vi "AssertVIExecCore.vi"(0 "VI Reference In":refnum<vi>, 1 "Label":string, 3 "Assert Only? (F)":bool, 5 "Execution:State":T2(array[ring]), 11 "Error In":errorcluster, 12 "Assert Interval(10 ms)":u32=10, 13 "Timeout(5 sec)":dbl=5.0) -> (4 "VI Reference Out":refnum<vi>, 6 "Asserted Value":T1(ring), 15 "Error Out":errorcluster)   [LabVIEW 2016, in "Drona.lvlib" / "AssertVI.lvlib"]
doc: "Asserts the execution state of the VI.\nThe input control name is given as a string , incase of path, use delimiters inbetween the path."
uses:
  AssertVI.lvlib
  <vilib>/addons/_JKI Toolkits/Caraya/classes/Assert/Assert True.vi
  <vilib>/addons/_JKI Toolkits/Caraya/classes/Assert/Assert.lvclass
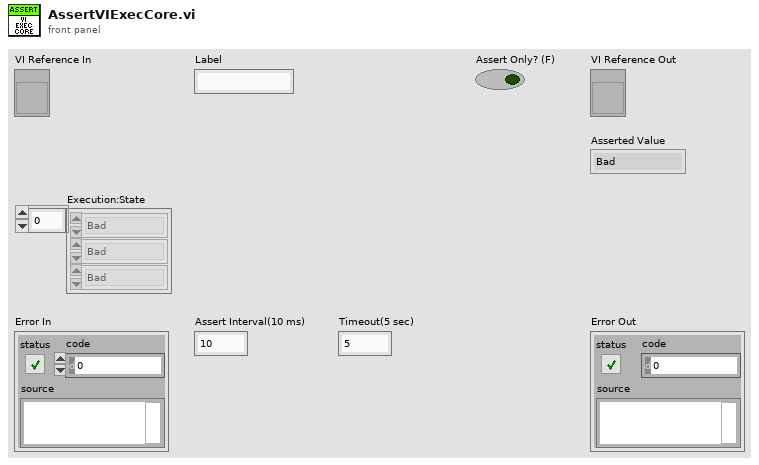
[diagram p1: front panel]
types:
  T1 = enum32{"Bad", "Idle", "Run top level", "Running"}
  T2 = enum32{"Bad", "Idle", "Run top level", "Running"}[]
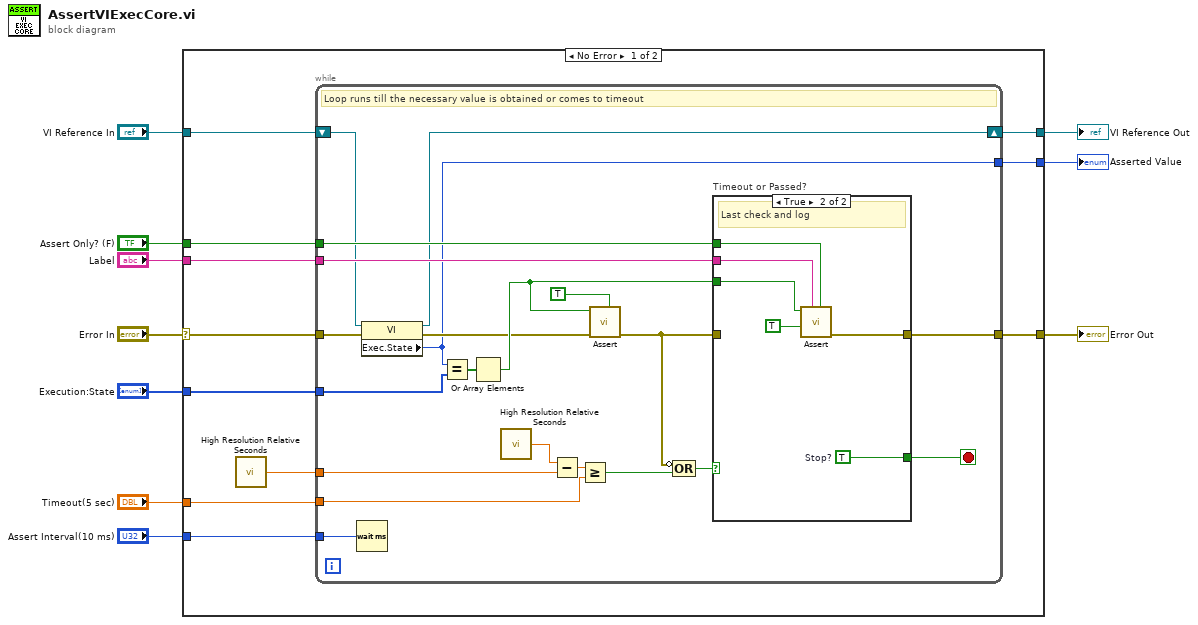
[diagram p0: block diagram]
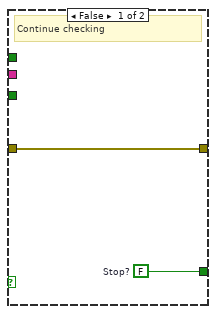
[diagram p2: hidden frame]
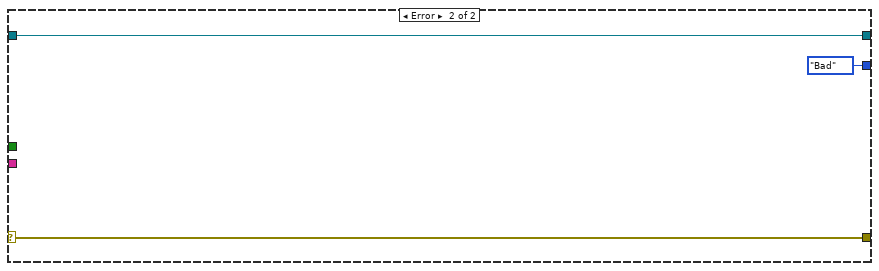
[diagram p3: hidden frame]
diagram:
  n1 = case shown="No Error" "Error In" {
    selector: "Error In" -> [w17 w53]
    tunnel: "Timeout(5 sec)" -> [w21 _]
    tunnel: [w20 w52] -> w9
    tunnel: [w12 w53] -> w8
    tunnel: "Assert Interval(10 ms)" -> [w19 _]
    tunnel: "Label" -> [w18 _]
    tunnel: "VI Reference In" -> [w16 w52]
    tunnel: "Assert Only? (F)" -> [w14 _]
    tunnel: "Execution:State" -> [w13 _]
    tunnel: [w11 T1."Bad" ("Exec.State")] -> w1
    frame No Error {
      n2 = call <vilib>:"High Resolution Relative Seconds.vi"() -> ("relative seconds"=w15:dbl)
      n3 = while {
        tunnel: w21 -> [w41]
        tunnel: w15 -> [w42]
        tunnel: w17 -> [w37]
        tunnel: [w39] -> w12
        tunnel: w19 -> [w38]
        tunnel: w18 -> [w36]
        shift-right: [w23] -> w20
        shift-left: w16 -> [w24]
        tunnel: w14 -> [w35]
        tunnel: w13 -> [w34]
        tunnel: [w22] -> w11
        stop <- w40 stop-if-true
        # "Loop runs till the necessary value is obtained or comes to timeout"
        n4 = Wait (ms)(milliseconds to wait=w38) -> ()  [unwired: 1 out]
        n5 = property class="VI"(reference=w24, error in=w37) -> (reference out=w23:refnum<vi>, error out=w25:errorcluster, "Exec.State"=w22:T1)
        n6 = Equal?(x=w22, y=w34) -> (x = y?=w27:bool[])
        n7 = Or Array Elements(Boolean array=w27) -> (logical OR=w26:bool)
        n8 = call <vilib>:"High Resolution Relative Seconds.vi"() -> ("relative seconds"=w33:dbl)
        n9 = Subtract(x=w33, y=w42) -> (x-y=w32:dbl)
        n10 = Greater Or Equal?(x=w32, y=w41) -> (x >= y?=w31:bool)
        n11 = call-poly <vilib>:"Assert.vi"("Assert Only? (F)"=TRUE, "error in (no error)"=w25, "True?"=w26) -> ("error out"=w30:errorcluster)  [unwired: 7 in, 1 out]
        n12 = Compound Arithmetic op=OR(invert w30, w31) -> (w29:bool)
        n13 = case "Timeout or Passed?" shown="True" w29 {
          tunnel: w30 -> [w44 _]
          tunnel: w26 -> [_ w49]
          tunnel: w36 -> [_ w50]
          tunnel: [w44 w48] -> w39
          tunnel: [w43 w47] -> w40
          tunnel: w35 -> [_ w45]
          frame False {
            w43 = FALSE  # Stop?
            # "Continue checking"
          }
          frame True {
            w47 = TRUE  # Stop?
            # "Last check and log"
            n14 = call-poly <vilib>:"Assert.vi"("Assert Only? (F)"=w45, "Label"=w50, "Register with caller test (F)"=TRUE, "True?"=w49) -> ("error out"=w48:errorcluster)  [unwired: 6 in, 1 out]
          }
        }
      }
    }
    frame Error {
    }
  }
  "Error Out" <- w8
  "VI Reference Out" <- w9
  "Asserted Value" <- w1
